vi "WaveformGeneration.vi"() -> ()   [LabVIEW 2020]
panel:
  out "Awg freq (MHz) 7":dbl
  out "Awg freq (MHz) 6":dbl
  out "Awg freq (MHz) 5":dbl
  out "Awg freq (MHz) 4":dbl
  out "Awg freq (MHz) 3":dbl
  out "Awg freq (MHz) 2":dbl
  in  "Path":path
  out "Waveform Graph":i16[](graph)
  out "size(s)":i32
  out "Awg freq (MHz)":dbl
  out "s? t:f":dbl
  in  "Phase 7":dbl caption="Phase"
  in  "Amplitude 7":dbl caption="Amplitude"
  in  "Frequency 7":dbl=316.621 caption="Frequency"
  in  "Phase 6":dbl caption="Phase"
  in  "Amplitude 6":dbl caption="Amplitude"
  in  "Frequency 6":dbl=312.934 caption="Frequency"
  in  "Phase 5":dbl caption="Phase"
  in  "Amplitude 5":dbl caption="Amplitude"
  in  "Frequency 5":dbl=309.248 caption="Frequency"
  in  "Phase 4":dbl caption="Phase"
  in  "Amplitude 4":dbl caption="Amplitude"
  in  "Frequency 4":dbl=305.55 caption="Frequency"
  in  "Phase 3":dbl caption="Phase"
  in  "Amplitude 3":dbl caption="Amplitude"
  in  "Frequency 3":dbl=301.875 caption="Frequency"
  in  "Phase 2":dbl caption="Phase"
  in  "Amplitude 2":dbl caption="Amplitude"
  in  "Frequency 2":dbl=298.19 caption="Frequency"
  in  "Phase":dbl
  in  "Amplitude":dbl=1.0
  in  "Frequency":dbl=294.502
  out "Array":i16[](array[numeric])
  in  "Data Length":i16
  out "appended path":path
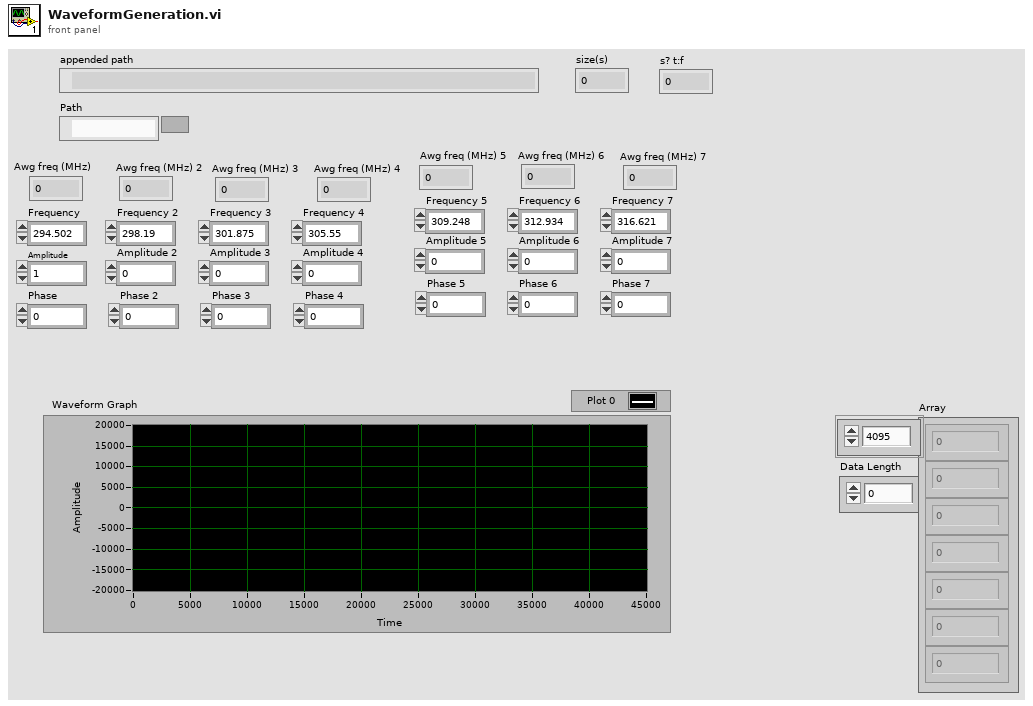
[diagram p1: front panel]
types:
  T1 = enum16{"big-endian, network order", "native, host order", "little-endian"}
  T2 = enum16{"open", "replace", "create", "open or create", "replace or create", "replace or create with confirmation"}
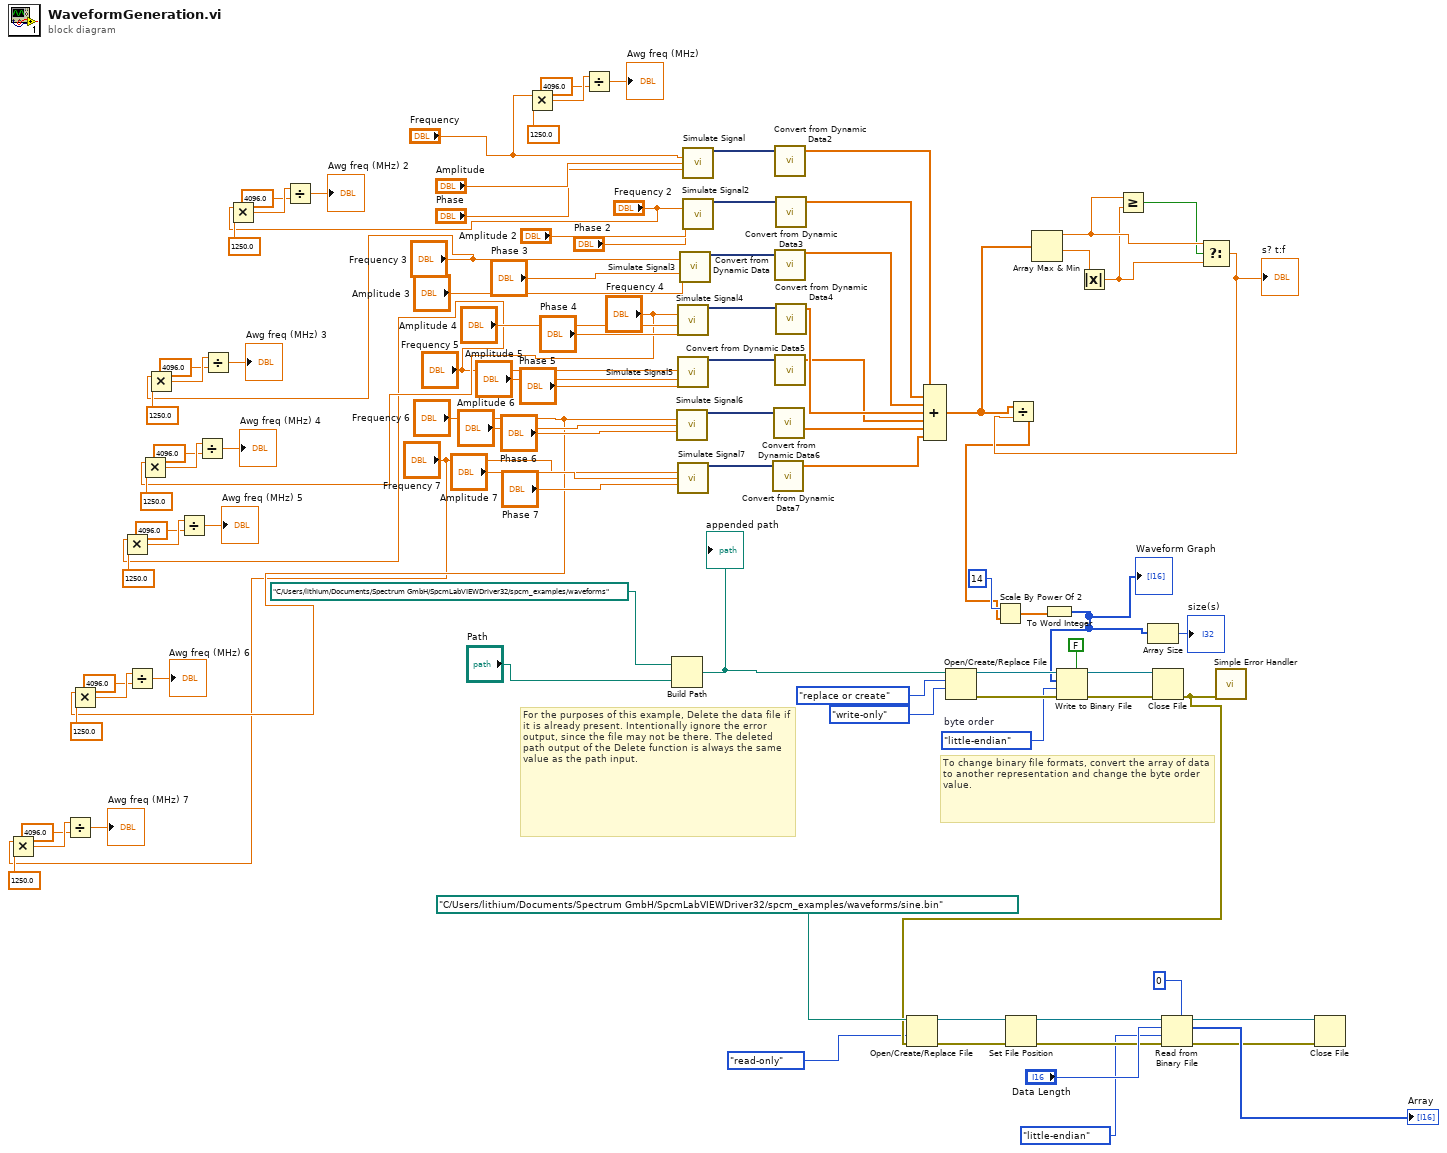
[diagram p0: block diagram]
diagram:
  w92 = T1."little-endian"  # byte order
  # "To change binary file formats, convert the array of data to another representation and change the byte order value."
  # "For the purposes of this example, Delete the data file if it is already present. Intentionally ignore the error output, since the file may not be there. The deleted path output of the Delete function is always the same value as the path input."
  n1 = Multiply(x="Frequency 7", y=1250.0) -> (x*y=w4:dbl)
  n2 = Divide(x=w4, y=4096.0) -> (x/y=→"Awg freq (MHz) 7":dbl)
  n3 = Multiply(x="Frequency 6", y=1250.0) -> (x*y=w9:dbl)
  n4 = Multiply(x="Frequency 5", y=1250.0) -> (x*y=w14:dbl)
  n5 = Divide(x=w9, y=4096.0) -> (x/y=→"Awg freq (MHz) 6":dbl)
  n6 = Multiply(x="Frequency 4", y=1250.0) -> (x*y=w19:dbl)
  n7 = Multiply(x="Frequency 3", y=1250.0) -> (x*y=w24:dbl)
  n8 = Divide(x=w14, y=4096.0) -> (x/y=→"Awg freq (MHz) 5":dbl)
  n9 = Divide(x=w19, y=4096.0) -> (x/y=→"Awg freq (MHz) 4":dbl)
  n10 = Divide(x=w24, y=4096.0) -> (x/y=→"Awg freq (MHz) 3":dbl)
  n11 = Multiply(x="Frequency 2", y=1250.0) -> (x*y=w29:dbl)
  n12 = Divide(x=w29, y=4096.0) -> (x/y=→"Awg freq (MHz) 2":dbl)
  n13 = Multiply(x="Frequency", y=1250.0) -> (x*y=w37:dbl)
  n14 = Divide(x=w37, y=4096.0) -> (x/y=→"Awg freq (MHz)":dbl)
  n15 = Build Path(base path=path "C:/Users/lithium/Documents/Spectrum GmbH/SpcmLabVIEWDriver32/spcm_examples/waveforms", name or relative path="Path") -> (appended path=w34:path)
  "appended path" <- w34
  n16 = call "Simulate Signal6"("Frequency"="Frequency 6", "Amplitude"="Amplitude 6", "Phase"="Phase 6") -> ("Sine"=w74:dynamicdata)  [unwired: 11 in, 1 out]
  n17 = call "Simulate Signal4"("Frequency"="Frequency 4", "Amplitude"="Amplitude 4", "Phase"="Phase 4") -> ("Sine"=w68:dynamicdata)  [unwired: 11 in, 1 out]
  n18 = call "Simulate Signal5"("Frequency"="Frequency 5", "Amplitude"="Amplitude 5", "Phase"="Phase 5") -> ("Sine"=w72:dynamicdata)  [unwired: 11 in, 1 out]
  n19 = call "Simulate Signal7"("Frequency"="Frequency 7", "Amplitude"="Amplitude 7", "Phase"="Phase 7") -> ("Sine"=w73:dynamicdata)  [unwired: 11 in, 1 out]
  n20 = call "Simulate Signal3"("Frequency"="Frequency 3", "Amplitude"="Amplitude 3", "Phase"="Phase 3") -> ("Sine"=w69:dynamicdata)  [unwired: 11 in, 1 out]
  n21 = call "Simulate Signal"("Frequency"="Frequency", "Amplitude"="Amplitude", "Phase"="Phase") -> ("Sine"=w71:dynamicdata)  [unwired: 11 in, 1 out]
  n22 = call "Simulate Signal2"("Frequency"="Frequency 2", "Amplitude"="Amplitude 2", "Phase"="Phase 2") -> ("Sine"=w70:dynamicdata)  [unwired: 11 in, 1 out]
  n23 = call "Convert from Dynamic Data7"("Dynamic Data Type"=w73) -> ("Array"=w61:dbl[])  [unwired: 3 in]
  n24 = call "Convert from Dynamic Data6"("Dynamic Data Type"=w74) -> ("Array"=w62:dbl[])  [unwired: 3 in]
  n25 = call "Convert from Dynamic Data2"("Dynamic Data Type"=w71) -> ("Array"=w67:dbl[])  [unwired: 3 in]
  n26 = call "Convert from Dynamic Data"("Dynamic Data Type"=w69) -> ("Array"=w65:dbl[])  [unwired: 3 in]
  n27 = call "Convert from Dynamic Data5"("Dynamic Data Type"=w72) -> ("Array"=w63:dbl[])  [unwired: 3 in]
  n28 = call "Convert from Dynamic Data3"("Dynamic Data Type"=w70) -> ("Array"=w66:dbl[])  [unwired: 3 in]
  n29 = call "Convert from Dynamic Data4"("Dynamic Data Type"=w68) -> ("Array"=w64:dbl[])  [unwired: 3 in]
  n30 = Compound Arithmetic op=ADD(w67, w66, w65, w64, w63, w62, w61) -> (w56:dbl[])
  n31 = Open/Create/Replace File(file path (use dialog)=w34, operation (0:open)=T2."replace or create", access (0:read/write)=enum16{"read/write", "read-only", "write-only"}."write-only") -> (refnum out=w95:refnum<file>, error out=w96:errorcluster)  [unwired: 3 in, 1 out]
  n32 = Array Max & Min(array=w56) -> (max value=w59:dbl, min value=w60:dbl)  [unwired: 2 out]
  n33 = Absolute Value(x=w60) -> (abs(x)=w58:dbl)
  n34 = Greater Or Equal?(x=w59, y=w58) -> (x >= y?=w57:bool)
  n35 = Select(t=w59, s=w57, f=w58) -> (s? t:f=w55:dbl)
  "s? t:f" <- w55
  n36 = Divide(x=w56, y=w55) -> (x/y=w54:dbl[])
  n37 = Scale By Power Of 2(n=i16 14, x=w54) -> (x*2^n=w90:dbl[])
  n38 = To Word Integer(number=w90) -> (16bit integer=w32:i16[])
  "Waveform Graph" <- w32
  n39 = Write to Binary File(file (use dialog)=w95, data=w32, error in=w96, 5:FALSE ("prepend array or string size? (T)"), 9:w92) -> (refnum out=w98:refnum<file>, error out=w97:errorcluster)  [unwired: 1 in, 1 out]
  n40 = Array Size(array=w32) -> (size(s)=→"size(s)":i32)
  n41 = Close File(refnum=w98, error in=w97) -> (error out=w81:errorcluster)  [unwired: 1 out]
  n42 = Open/Create/Replace File(file path (use dialog)=path "C:/Users/lithium/Documents/Spectrum GmbH/SpcmLabVIEWDriver32/spcm_examples/waveforms/sine.bin", error in=w81, access (0:read/write)=enum16{"read/write", "read-only", "write-only"}."read-only") -> (refnum out=w84:refnum<file>, error out=w80:errorcluster)  [unwired: 3 in, 1 out]
  n43 = Set File Position(refnum=w84, error in=w80) -> (refnum out=w83:refnum<file>, error out=w79:errorcluster)  [unwired: 2 in]
  n44 = Read from Binary File(5:i16 0, 8:w79, 9:T1."little-endian" ("byte order (0:big-endian, network order)"), 10:"Data Length", 11:w83) -> (0:w78:errorcluster, 2:→"Array":i16[], 3:w86:refnum<file>)  [unwired: 1 in, 1 out]
  n45 = call <vilib>:"Simple Error Handler.vi"("error in (no error)"=w81) -> ()  [unwired: 4 in, 5 out]
  n46 = Close File(refnum=w86, error in=w78) -> ()  [unwired: 2 out]
